vi "Shutdown HW.vi"(8 "error in (no error)":errorcluster, 11 "DAQmx Servo in":refnum<class "DAQmx Servo.lvclass">) -> (0 "error out":errorcluster, 3 "DAQmx Servo out":refnum<class "DAQmx Servo.lvclass">)   [LabVIEW 2020, in "DAQmx Servo.lvclass"]
uses:
  DAQmx Servo.lvclass
  DAQmx Servo.lvclass/DAQmx Servo.ctl
  Servo.lvclass
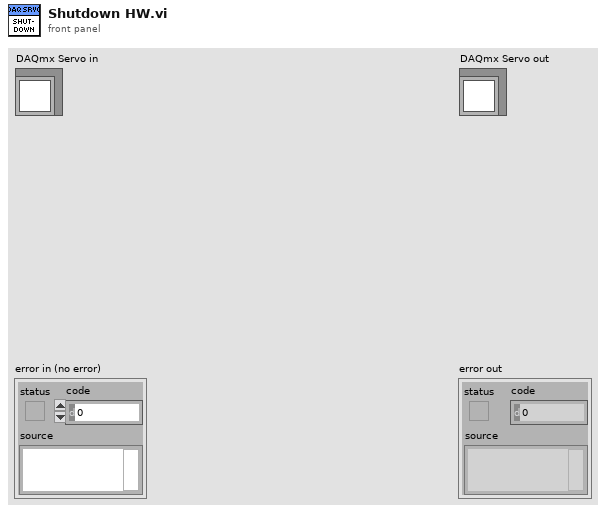
[diagram p1: front panel]
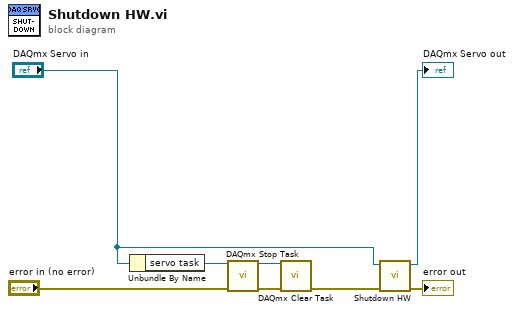
[diagram p0: block diagram]
diagram:
  n1 = Unbundle By Name("DAQmx Servo in") -> ("servo task"=w3:refnum<k21>)
  n2 = call <vilib>:"DAQmx Stop Task.vi"("task/channels in"=w3, "error in"="error in (no error)") -> ("task out"=w2:refnum<k21>, "error out"=w6:errorcluster)  [unwired: 12 in]
  n3 = call <vilib>:"DAQmx Clear Task.vi"("task in"=w2, "error in"=w6) -> ("error out"=w4:errorcluster)  [unwired: 13 in]
  n4 = call-parent "Shutdown HW.vi"("error in (no error)"=w4, "Servo in"="DAQmx Servo in") -> ("error out"=→"error out":errorcluster, "Servo out"=→"DAQmx Servo out":refnum<class "DAQmx Servo.lvclass">)  [unwired: 8 in]
